vi "BK Precision 9103 Output DC Volts.vi"() -> ()   [LabVIEW 2022 SP3]
doc: "This example shows how to configure the instrument's output voltage level, over current protection, and over voltage protection. The actual voltage level and actual current level are returned as well as whether over voltage protection (OVP) or over current protection (OCP) has been tripped."
uses:
  <instrlib>/BK Precision 9103/BK Precision 9103.lvlib
panel:
  in  "Preset (1)":i32(ring) items=["Preset1", "Preset2", "Preset3", "Normal Mode"]
  out "CC/CV model":bool
  out "Displayed Voltage Value":dbl format="%.2g"
  out "Displayed Current Value":dbl format="%.1g"
  in  "Voltage Level (0.0 V)":dbl format="%.2g"
  in  "Current Limit (0.0 A)":dbl format="%.2g"
  in  "Serial Configuration":T1={"Baud Rate"=9600, "Parity"=0, "Data Bits"=8, "Stop Bits"=10, "Flow Control"=0} {"Flow Control" items=["None", "XON/XOFF", "RTS/CTS", "XON/XOFF & RTS/CTS", "DTR/DSR", "XON/XOFF & DTR/DSR"]; "Stop Bits" items=["1.0"=10, "1.5"=15, "2.0"=20]; "Data Bits" items=["7"=7, "8"=8]; "Parity" items=["None", "Odd", "Even", "Mark", "Space"]; "Baud Rate" items=["300"=300, "600"=600, "1200"=1200, "2400"=2400, "4800"=4800, "9600"=9600, "19200"=19200]}
  in  "Stop Output":bool
  in  "VISA resource name":refnum<visa-resource-name>
  # "(c) 2014 <BK Precision>.  ALL RIGHTS RESERVED."
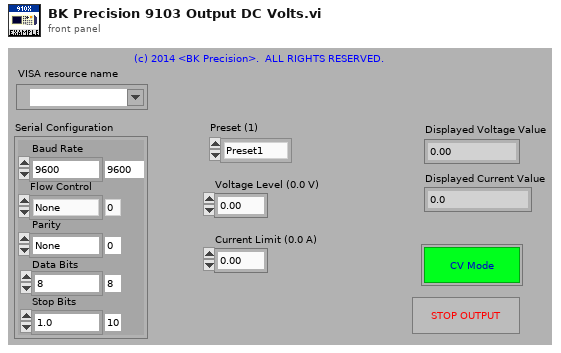
[diagram p1: front panel]
types:
  T1 = cluster{"Baud Rate":u32, "Parity":u16, "Data Bits":u16, "Stop Bits":u16, "Flow Control":u16}
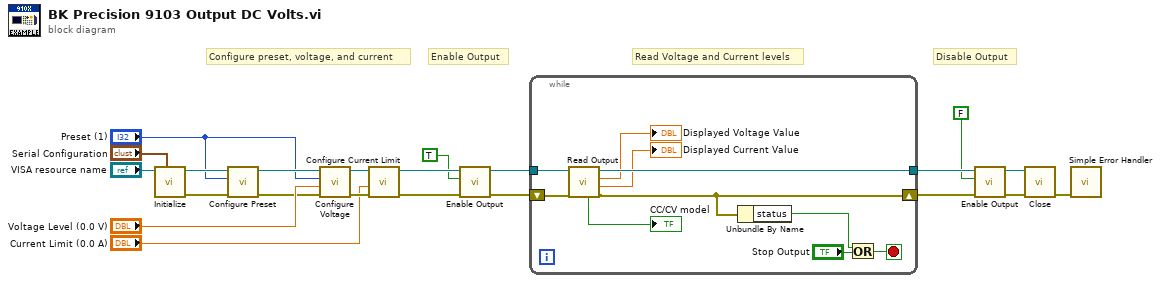
[diagram p0: block diagram]
diagram:
  # "Disable Output"
  # "Read Voltage and Current levels"
  # "Enable Output"
  # "Configure preset, voltage, and current"
  n1 = call <instrlib>:"Initialize.vi"("Serial Configuration"="Serial Configuration", "VISA resource name"="VISA resource name") -> ("error out"=w5:errorcluster, "VISA resource name out"=w6:refnum<visa-resource-name>)  [unwired: 8 in]
  n2 = call <instrlib>:"Configure Preset.vi"("error in (no error)"=w5, "Preset"="Preset (1)", "VISA resource name"=w6) -> ("error out"=w4:errorcluster, "VISA resource name out"=w3:refnum<visa-resource-name>)  [unwired: 7 in]
  n3 = call <instrlib>:"Configure Voltage.vi"("error in (no error)"=w4, "Voltage Level (0.0 V)"="Voltage Level (0.0 V)", "Preset"="Preset (1)", "VISA resource name"=w3) -> ("error out"=w17:errorcluster, "VISA resource name out"=w20:refnum<visa-resource-name>)  [unwired: 6 in]
  n4 = call <instrlib>:"Configure Current Limit.vi"("error in (no error)"=w17, "Current Limit (0.0 A)"="Current Limit (0.0 A)", "VISA resource name"=w20) -> ("error out"=w18:errorcluster, "VISA resource name out"=w19:refnum<visa-resource-name>)  [unwired: 7 in]
  n5 = call <instrlib>:"Enable Output.vi"("error in (no error)"=w18, "Enable Output (F: Disabled)"=TRUE, "VISA resource name"=w19) -> ("error out"=w16:errorcluster, "VISA resource name out"=w15:refnum<visa-resource-name>)  [unwired: 7 in]
  n6 = while {
    shift-right: [w27] -> w14
    shift-left: w16 -> [w29]
    tunnel: w15 -> [w28]
    tunnel: [w26] -> w13
    stop <- w32 stop-if-true
    n7 = call <instrlib>:"Read Output.vi"("error in (no error)"=w29, "VISA resource name"=w28) -> ("error out"=w27:errorcluster, "Displayed Current Value"=→"Displayed Current Value":dbl, "Displayed Voltage Value"=→"Displayed Voltage Value":dbl, "VISA resource name out"=w26:refnum<visa-resource-name>, "CC/CV model"=→"CC/CV model":bool)  [unwired: 5 in]
    n8 = Unbundle By Name(w27) -> ("status"=w30:bool)
    n9 = Or(x=w30, y="Stop Output") -> (x .or. y?=w32:bool)
  }
  n10 = call <instrlib>:"Enable Output.vi"("error in (no error)"=w14, "Enable Output (F: Disabled)"=FALSE ("Enable Output"), "VISA resource name"=w13) -> ("error out"=w10:errorcluster, "VISA resource name out"=w11:refnum<visa-resource-name>)  [unwired: 7 in]
  n11 = call <instrlib>:"Close.vi"("error in (no error)"=w10, "VISA resource name"=w11) -> ("error out"=w22:errorcluster)  [unwired: 9 in]
  n12 = call <vilib>:"Simple Error Handler.vi"("error in (no error)"=w22) -> ()  [unwired: 4 in, 5 out]
